vi "Stable Check.vi"(0 "Tolerance":dbl, 1 "AbsError":dbl, 2 "PI Running?":bool, 5 "ReqReads":i32, 7 "Parameter":i32, 9 "Setpoint":dbl format="%#_13g", 11 "StabilityCount In":i32) -> (4 "HalfTol":bool, 8 "Stable?":bool, 15 "StabilityCount Out":i32)   [LabVIEW 2013]
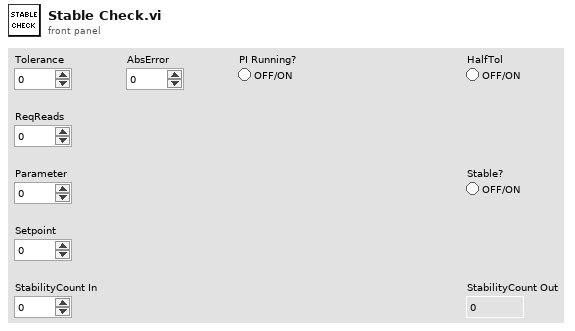
[diagram p1: front panel]
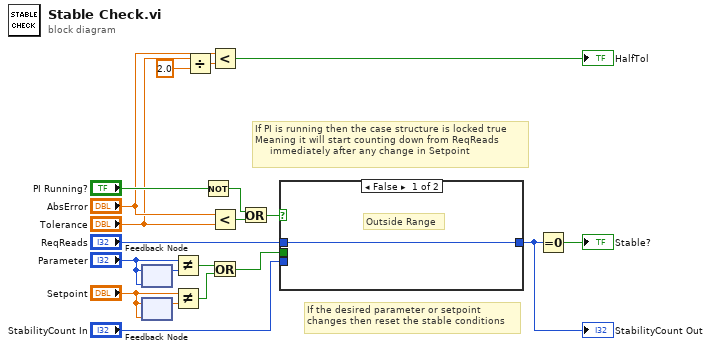
[diagram p0: block diagram]
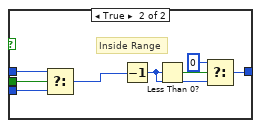
[diagram p2: hidden frame]
diagram:
  # "If PI is running then the case structure is locked true\nMeaning it will start counting down from ReqReads\n     immediately after any change in Setpoint"
  # "If the desired parameter or setpoint\nchanges then reset the stable conditions"
  n1 = feedback #1("Parameter") -> (w14:i32)
  n2 = feedback-in #1("Parameter") -> ()
  n3 = feedback #2("Setpoint") -> (w15:dbl)
  n4 = feedback-in #2("Setpoint") -> ()
  n5 = Not Equal?(x="Parameter", y=w14) -> (x != y?=w16:bool)
  n6 = Not Equal?(x="Setpoint", y=w15) -> (x != y?=w17:bool)
  n7 = Divide(x="Tolerance", y=2.0) -> (x/y=w4:dbl)
  n8 = Not(x="PI Running?") -> (.not. x?=w18:bool)
  n9 = Less?(x="AbsError", y=w4) -> (x < y?=→"HalfTol":bool)
  n10 = Less?(x="AbsError", y="Tolerance") -> (x < y?=w19:bool)
  n11 = Or(x=w16, y=w17) -> (x .or. y?=w13:bool)
  n12 = Or(x=w18, y=w19) -> (x .or. y?=w20:bool)
  n13 = case shown="False" w20 {
    tunnel: [w21 w26] -> w9
    tunnel: "ReqReads" -> [w21 w24]
    tunnel: w13 -> [_ w25]
    tunnel: "StabilityCount In" -> [_ w22]
    frame False {
      # "Outside Range"
    }
    frame True {
      # "Inside Range"
      n14 = Select(t=w24, s=w25, f=w22) -> (s? t:f=w23:i32)
      n15 = Decrement(x=w23) -> (x-1=w28:i32)
      n16 = Less Than 0?(x=w28) -> (x < 0?=w27:bool)
      n17 = Select(t=0, s=w27, f=w28) -> (s? t:f=w26:i32)
    }
  }
  "StabilityCount Out" <- w9
  n18 = Equal To 0?(x=w9) -> (x = 0?=→"Stable?":bool)
